vi "light ON and OFF.vi"() -> ()   [LabVIEW 2023]
panel:
  in  "stop":bool
  in  "Boolean 2":bool
  out "Boolean":bool
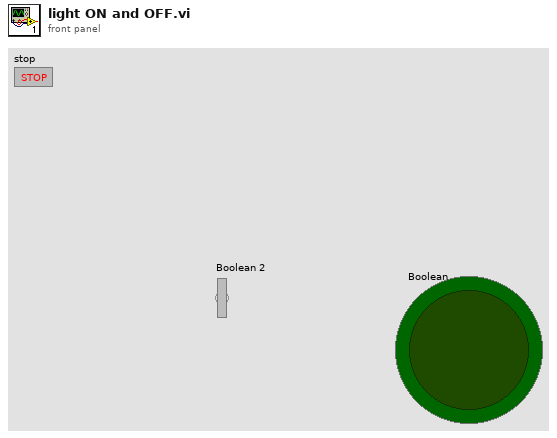
[diagram p1: front panel]
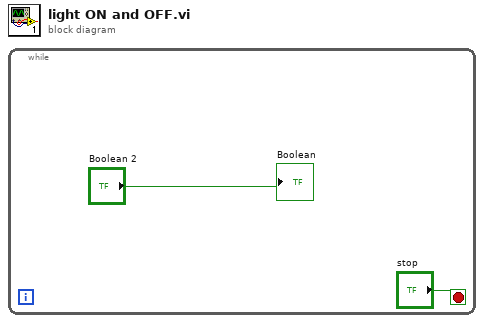
[diagram p0: block diagram]
diagram:
  n1 = while {
    stop <- "stop" stop-if-true
    "Boolean" <- "Boolean 2"
  }
